vi "SDCCB Device Engine.vi"(0 "SDCCB Notifier Name":string="Box01", 11 "COM Port":string[](array[string])) -> ()   [LabVIEW 2020]
uses:
  Spinning Disk Type Defs/SD Notifer Data.ctl
  Spinning Disk Type Defs/SD Actions.ctl
  <vilib>/Instr/_visa.llb/VISA Configure Serial Port (Instr).vi
panel:
  in  "Get All Positions":bool
  in  "Disk On":bool
  in  "Disk Position":i32=1 min=1 max=3
  out "Latest Error":errorcluster
  in  "Quit":bool
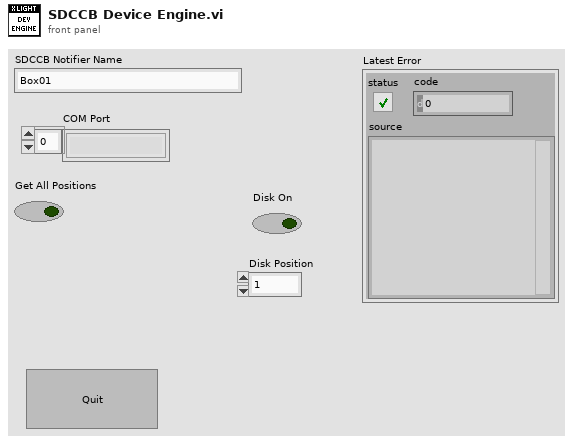
[diagram p1: front panel]
types:
  T1 = typedef "SD Notifer Data.ctl" = cluster{"Actions":T2, "Disk On?":bool, "Dichroic Pos.":i32, "Filter Wheel Pos.":i32, "Disk Pos.":i32, "Recived":bool, "Num Pos":i32[]}
  T2 = typedef "SD Actions.ctl" = enum16{"Status", "Get All Pos.", "Get Num. Pos.", "Home All", "Set Filter Wheel Pos.", "Set Disk Pos.", "Set Dichroic Pos.", "Disk On", "Disk Off", "Quit"}
  T3 = enum32{"Invalid", "Standard", "Closed", "Hidden", "Minimized", "Maximized"}
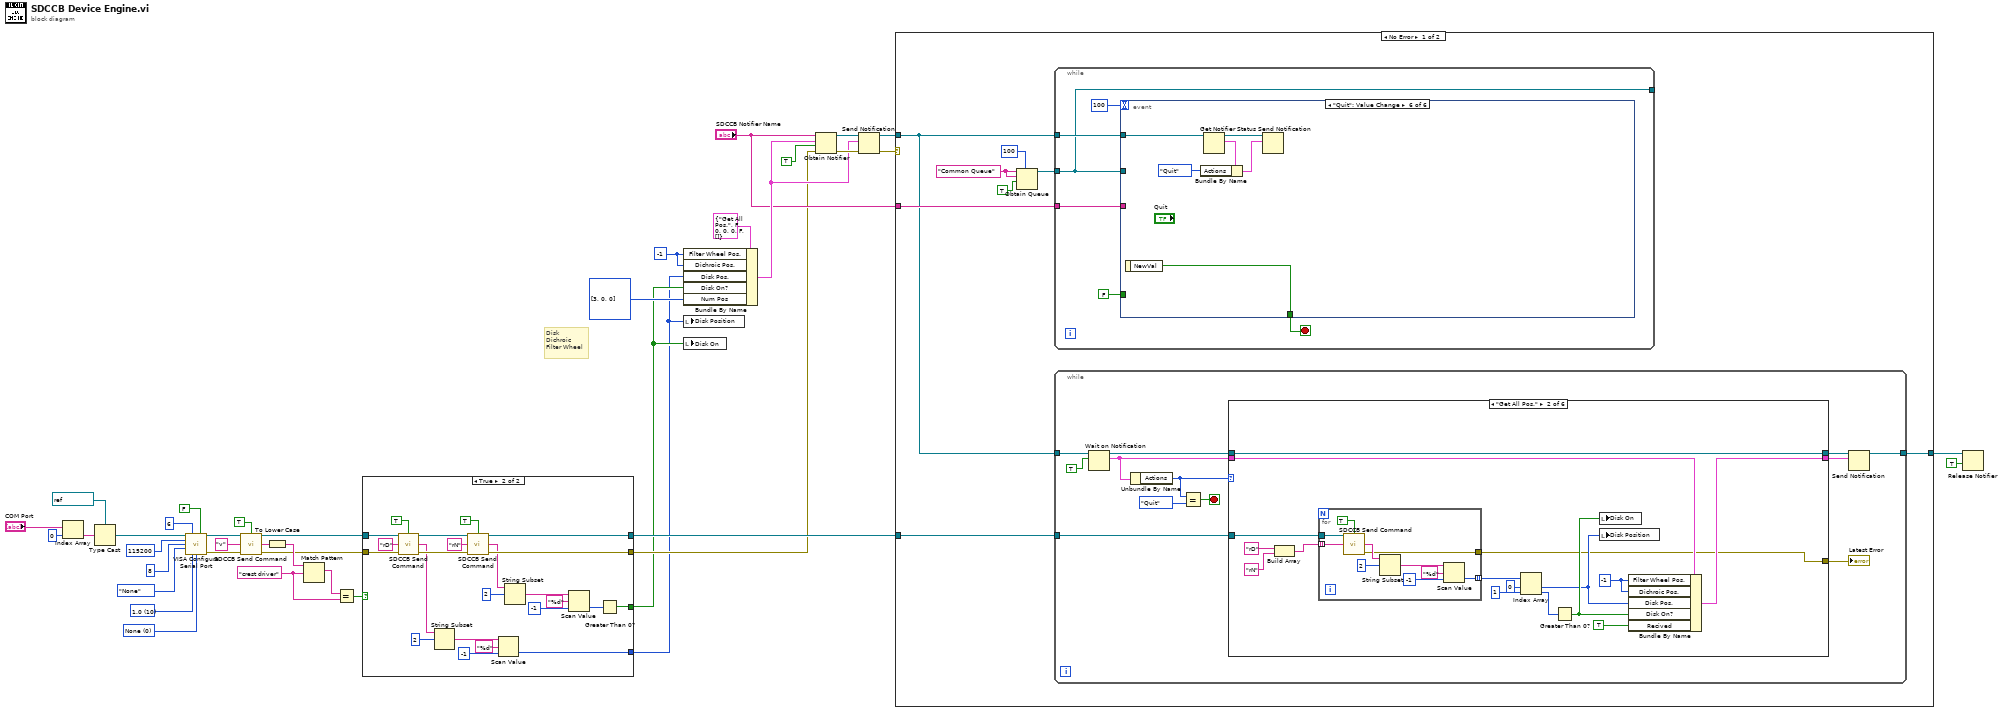
[diagram p0: block diagram]
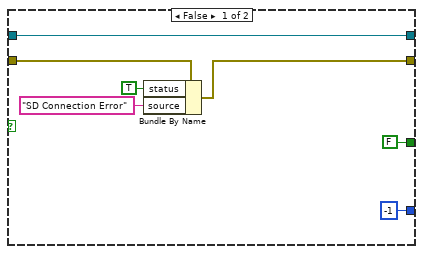
[diagram p2: hidden frame]
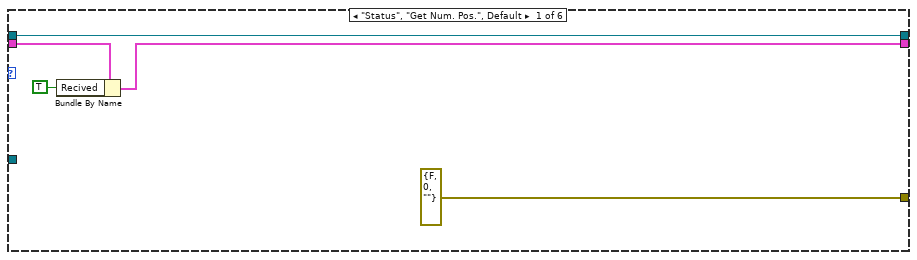
[diagram p3: hidden frame]
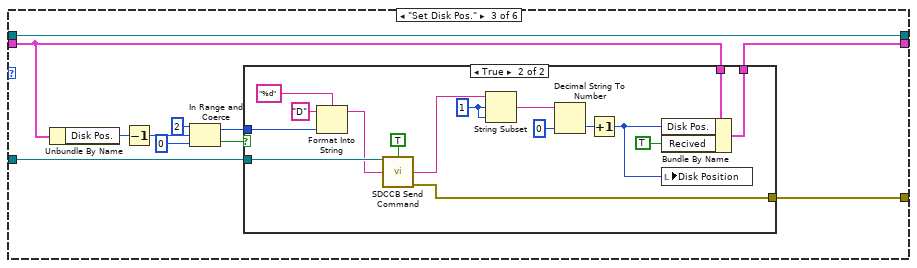
[diagram p4: hidden frame]
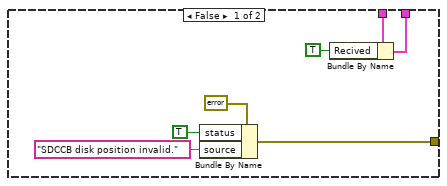
[diagram p5: hidden frame]
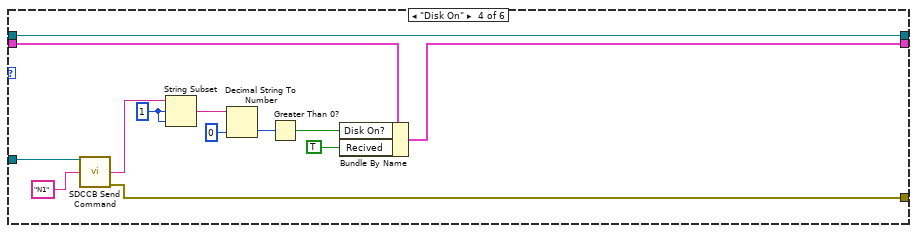
[diagram p6: hidden frame]
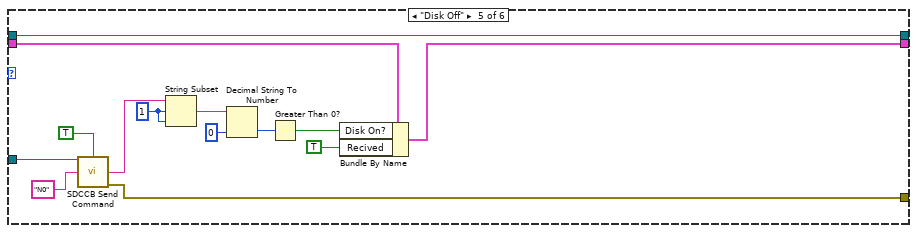
[diagram p7: hidden frame]
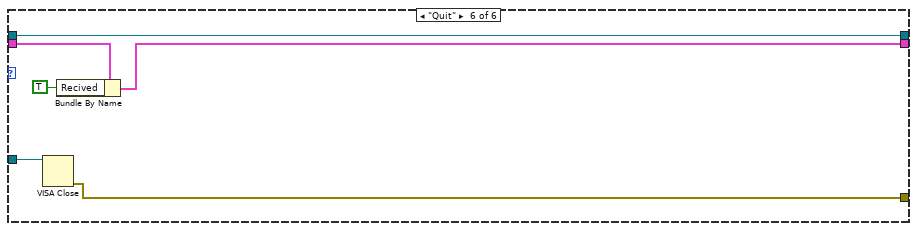
[diagram p8: hidden frame]
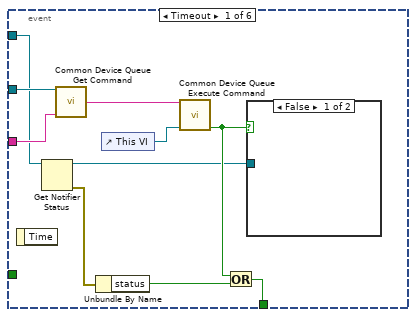
[diagram p9: hidden frame]
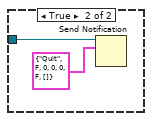
[diagram p10: hidden frame]
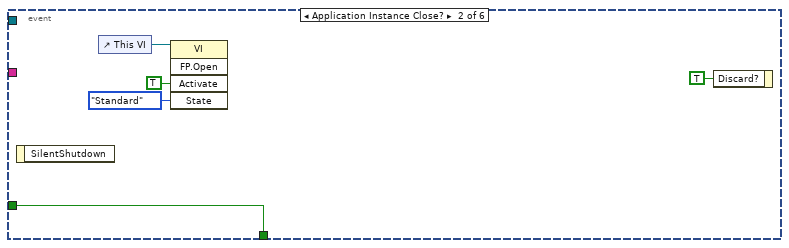
[diagram p11: hidden frame]
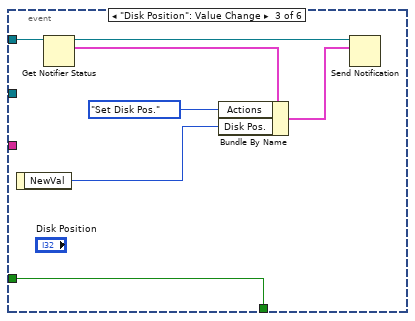
[diagram p12: hidden frame]
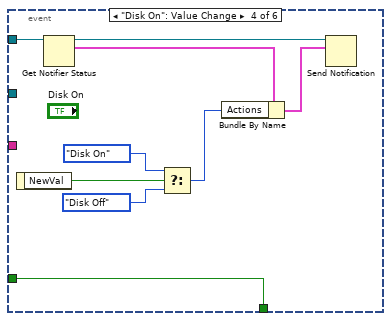
[diagram p13: hidden frame]
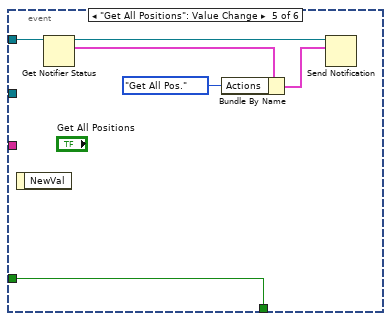
[diagram p14: hidden frame]
diagram:
  w10 = "crest driver"
  w13 = -1 ("Filter Wheel Pos.")
  w18 = u16 0 items=["None", "XON/XOFF", "RTS/CTS", "XON/XOFF & RTS/CTS", "DTR/DSR", "XON/XOFF & DTR/DSR"] ("flow control (0:none)")
  w19 = u16 10 items=["1.0"=10, "1.5"=15, "2.0"=20] ("stop bits (10: 1 bit)")
  # "Disk\nDichroic\nFilter Wheel"
  n1 = Index Array(array="COM Port", index=0) -> (element=w36:string)
  n2 = Type Cast(type=refnum<visa-resource-name> "COM5" ("VISA resource name"), x=w36) -> (*(type *) &x=w16:refnum<visa-resource-name>)
  n3 = call-poly "VISA Configure Serial Port"("VISA resource name"=w16, "timeout (10sec)"=u32 6, "Enable Termination\nChar (T)"=FALSE ("Enable Termination\nChar (T)"), "baud rate (9600)"=u32 115200, "data bits (8)"=u16 8, "parity (0:none)"=enum16{"None", "Odd", "Even", "Mark", "Space"}."None", "stop bits (10: 1 bit)"=w19, "flow control (0:none)"=w18) -> ("VISA resource name out"=w15:refnum<visa-resource-name>, "error out"=w14:errorcluster)  [unwired: 6 in]
  n4 = call "SDCCB Send Command.vi"("VISA Ref"=w15, "Wait for Reply (T)"=TRUE, "Command"="v", "Error In"=w14) -> ("VISA Ref Dup"=w6:refnum<visa-resource-name>, "Reply"=w9:string, "Error Out"=w7:errorcluster)  [unwired: 9 in]
  n5 = To Lower Case(string=w9) -> (all lower case string=w12:string)
  n6 = Match Pattern(string=w12, regular expression=w10) -> (match substring=w11:string)  [unwired: 1 in, 3 out]
  n7 = Equal?(x=w11, y=w10) -> (x = y?=w8:bool)
  n8 = case shown="True" w8 {
    tunnel: w7 -> [w46 w67]
    tunnel: [w43 w61] -> w3
    tunnel: w6 -> [w42 w69]
    tunnel: [w42 w49] -> w4
    tunnel: [FALSE w48] -> w2
    tunnel: [-1 ("default (0 dbl)") w47] -> w1
    frame False {
      n9 = Bundle By Name(cluster=w46, "status"=TRUE, "source"="SD Connection Error") -> (w43:errorcluster)
    }
    frame True {
      n10 = call "SDCCB Send Command.vi"("VISA Ref"=w69, "Wait for Reply (T)"=TRUE, "Command"="rD", "Error In"=w67) -> ("VISA Ref Dup"=w62:refnum<visa-resource-name>, "Reply"=w60:string, "Error Out"=w63:errorcluster)  [unwired: 9 in]
      n11 = String Subset(string=w60, offset (0)=2) -> (substring=w58:string)  [unwired: 1 in]
      n12 = call "SDCCB Send Command.vi"("VISA Ref"=w62, "Wait for Reply (T)"=TRUE, "Command"="rN", "Error In"=w63) -> ("VISA Ref Dup"=w49:refnum<visa-resource-name>, "Reply"=w51:string, "Error Out"=w61:errorcluster)  [unwired: 9 in]
      n13 = Scan Value(string=w58, format string="%d", default (0 dbl)=-1) -> (value=w47:i32)  [unwired: 1 out]
      n14 = String Subset(string=w51, offset (0)=2) -> (substring=w53:string)  [unwired: 1 in]
      n15 = Scan Value(string=w53, format string="%d", default (0 dbl)=-1) -> (value=w50:i32)  [unwired: 1 out]
      n16 = Greater Than 0?(x=w50) -> (x > 0?=w48:bool)
    }
  }
  n17 = Bundle By Name(cluster=T1 {"Actions"=enum."Get All Pos.", "Disk On?"=FALSE, "Dichroic Pos."=0, "Filter Wheel Pos."=0, "Disk Pos."=0, "Recived"=FALSE, "Num Pos"=[]} ("XLight Notifier Data"), "Filter Wheel Pos."=w13, "Dichroic Pos."=w13, "Disk Pos."=w1, "Disk On?"=w2, "Num Pos"=i32[] [3, 0, 0]) -> (w30:T1)
  n18 = local write "Disk Position"(w1) -> ()
  n19 = local write "Disk On"(w2) -> ()
  n20 = Obtain Notifier(name (unnamed)="SDCCB Notifier Name", notification data type=w30, create if not found? (T)=TRUE, error in (no error)=w3) -> (notifier out=w34:refnum<notifier>, error out=w33:errorcluster)  [unwired: 1 out]
  n21 = Send Notification(notification=w30, notifier=w34, error in (no error)=w33) -> (notifier out=w28:refnum<notifier>, error out=w29:errorcluster)
  n22 = case shown="No Error" w29 {
    tunnel: w28 -> [w71 w239]
    tunnel: w4 -> [w72 _]
    tunnel: "SDCCB Notifier Name" -> [w77 _]
    tunnel: [w70 w239] -> w26
    frame No Error {
      w76 = "Common Queue" ("Unique Notifier Name")
      n23 = Obtain Queue(max queue size (-1, unlimited)=100, name (unnamed)=w76, element data type=w76, create if not found? (T)=TRUE) -> (queue out=w73:refnum<queue>)  [unwired: 1 in, 2 out]
      n24 = while {
        tunnel: w73 -> [w188]
        tunnel: w77 -> [w191]
        tunnel: w71 -> [w192]
        tunnel: [w188] -> _
        stop <- w190 stop-if-true
        # "ProScan 3 GUI and Common Queue Loop"
        n25 = event shown="[5] \"Quit\": Value Change" {
          selector: _ -> [_ _ _ _ _ _]
          dyn-events: _ -> [_ _ _ _ _ _]
          timeout: 100 -> [_ _ _ _ _ _]
          tunnel: w188 -> [w197 _ _ _ _ _]
          tunnel: w192 -> [w194 _ w216 w225 w231 w237]
          tunnel: w191 -> [w196 _ _ _ _ _]
          tunnel: [w195 w210 w217 w226 w232 w238] -> w190
          tunnel: FALSE -> [_ w210 w217 w226 w232 _]
          event Timeout {
            n26 = event-data() -> ()  [unwired: 1 in, 1 out]
            n27 = Get Notifier Status(notifier=w194) -> (notifier out=w198:refnum<notifier>, error out=w203:errorcluster)  [unwired: 1 in, 3 out]
            n28 = call "Common Device Queue Get Command.vi"("Common Queue"=w197, "Notifier Name"=w196) -> ("Command"=w202:string)  [unwired: 12 in, 1 out]
            n29 = Unbundle By Name(w203) -> ("status"=w200:bool)
            n30 = control-ref of="This VI"() -> (w201:refnum<vi>)
            n31 = call "Common Device Queue Execute Command.vi"("Common Command"=w202, "VI Refnum"=w201) -> ("Quit?"=w199:bool)  [unwired: 12 in, 1 out]
            n32 = Or(x=w199, y=w200) -> (x .or. y?=w195:bool)
            n33 = case shown="False" w199 {
              tunnel: w198 -> [_ w205]
              frame False {
              }
              frame True {
                n34 = Send Notification(notification=T1 {"Actions"=enum."Quit", "Disk On?"=FALSE, "Dichroic Pos."=0, "Filter Wheel Pos."=0, "Disk Pos."=0, "Recived"=FALSE, "Num Pos"=[]} ("XLight Notifier Data"), notifier=w205) -> ()  [unwired: 1 in, 2 out]
              }
            }
          }
          event Application Instance Close? {
            n35 = event-data() -> ()  [unwired: 1 in, 1 out]
            n36 = control-ref of="This VI"() -> (w207:refnum<vi>)
            n37 = invoke class="VI" method="FP.Open"(reference=w207, "Activate"=TRUE ("Activate?"), "State"=T3."Standard") -> ()  [unwired: 2 in, 5 out]
            n38 = event-data("Discard?"=TRUE) -> ()  [unwired: 1 in, 1 out]
          }
          event "Disk Position": Value Change {
            n39 = event-data() -> ("NewVal"=w212:i32)  [unwired: 1 in]
            n40 = Get Notifier Status(notifier=w216) -> (notifier out=w215:refnum<notifier>, current notification=w214:T1)  [unwired: 1 in, 3 out]
            n41 = Bundle By Name(cluster=w214, "Actions"=SD_Actions."Set Disk Pos.", "Disk Pos."=w212) -> (w211:T1)
            n42 = Send Notification(notification=w211, notifier=w215) -> ()  [unwired: 1 in, 2 out]
          }
          event "Disk On": Value Change {
            n43 = event-data() -> ("NewVal"=w221:bool)  [unwired: 1 in]
            n44 = Get Notifier Status(notifier=w225) -> (notifier out=w224:refnum<notifier>, current notification=w223:T1)  [unwired: 1 in, 3 out]
            n45 = Select(t=SD_Actions."Disk On" ("Actions"), s=w221, f=SD_Actions."Disk Off" ("Actions")) -> (s? t:f=w218:T2)
            n46 = Bundle By Name(cluster=w223, "Actions"=w218) -> (w222:T1)
            n47 = Send Notification(notification=w222, notifier=w224) -> ()  [unwired: 1 in, 2 out]
          }
          event "Get All Positions": Value Change {
            n48 = event-data() -> ()  [unwired: 1 in, 1 out]
            n49 = Get Notifier Status(notifier=w231) -> (notifier out=w230:refnum<notifier>, current notification=w229:T1)  [unwired: 1 in, 3 out]
            n50 = Bundle By Name(cluster=w229, "Actions"=SD_Actions."Get All Pos.") -> (w228:T1)
            n51 = Send Notification(notification=w228, notifier=w230) -> ()  [unwired: 1 in, 2 out]
          }
          event "Quit": Value Change {
            n52 = event-data() -> ("NewVal"=w238:bool)  [unwired: 1 in]
            n53 = Get Notifier Status(notifier=w237) -> (notifier out=w234:refnum<notifier>, current notification=w236:T1)  [unwired: 1 in, 3 out]
            n54 = Bundle By Name(cluster=w236, "Actions"=SD_Actions."Quit") -> (w233:T1)
            n55 = Send Notification(notification=w233, notifier=w234) -> ()  [unwired: 1 in, 2 out]
          }
        }
      }
      n56 = while {
        tunnel: w72 -> [w80]
        tunnel: w71 -> [w89]
        tunnel: [w78] -> w70
        stop <- w86 stop-if-true
        n57 = Wait on Notification(notifier=w89, ignore previous (F)=TRUE) -> (notifier out=w84:refnum<notifier>, notification=w83:T1)  [unwired: 2 in, 2 out]
        n58 = Unbundle By Name(w83) -> ("Actions"=w85:T2)
        n59 = Equal?(x=w85, y=SD_Actions."Quit") -> (x = y?=w86:bool)
        n60 = case shown="\"Get All Pos.\"" w85 {
          tunnel: w84 -> [w94 w110 w131 w167 w181 w187]
          tunnel: w83 -> [w93 w109 w128 w164 w178 w186]
          tunnel: [w94 w110 w131 w167 w181 w187] -> w82
          tunnel: [w91 w107 w127 w158 w172 w184] -> w81
          tunnel: w80 -> [_ w102 w130 w166 w180 w183]
          tunnel: [errorcluster {"status"=FALSE, "code"=0, "source"=""} ("Error Out") w95 w129 w165 w179 w182] -> w79
          frame "Status", "Get Num. Pos.", Default {
            n61 = Bundle By Name(cluster=w93, "Recived"=TRUE) -> (w91:T1)
          }
          frame "Get All Pos." {
            w106 = -1 ("Filter Wheel Pos.")
            n62 = Build Array("rD" ("Command"), "rN" ("Command")) -> (w105:string[])
            n63 = for {
              tunnel: [w114] -> w101 mode=indexing
              tunnel: w105 -> [w113] mode=indexing
              tunnel: w102 -> [w112]
              tunnel: [w111] -> w95
              n64 = call "SDCCB Send Command.vi"("VISA Ref"=w112, "Wait for Reply (T)"=TRUE, "Command"=w113) -> ("Reply"=w119:string, "Error Out"=w111:errorcluster)  [unwired: 10 in, 1 out]
              n65 = String Subset(string=w119, offset (0)=2) -> (substring=w117:string)  [unwired: 1 in]
              n66 = Scan Value(string=w117, format string="%d", default (0 dbl)=-1) -> (value=w114:i32)  [unwired: 1 out]
            }
            n67 = Index Array(array=w101, index #1=0 ("index"), index #2=1 ("index")) -> (element #1=w96:i32, element #2=w98:i32)
            n68 = Greater Than 0?(x=w98) -> (x > 0?=w97:bool)
            n69 = local write "Disk On"(w97) -> ()
            n70 = local write "Disk Position"(w96) -> ()
            n71 = Bundle By Name(cluster=w109, "Filter Wheel Pos."=w106, "Dichroic Pos."=w106, "Disk Pos."=w96, "Disk On?"=w97, "Recived"=TRUE) -> (w107:T1)
          }
          frame "Set Disk Pos." {
            n72 = Unbundle By Name(w128) -> ("Disk Pos."=w126:i32)
            n73 = Decrement(x=w126) -> (x-1=w121:i32)
            n74 = In Range and Coerce(upper limit=2, x=w121, lower limit=0) -> (coerced(x)=w122:i32, In Range?=w123:bool)
            n75 = case shown="True" w123 {
              tunnel: w130 -> [_ w154]
              tunnel: [w132 w153] -> w129
              tunnel: w128 -> [w137 w149]
              tunnel: [w136 w143] -> w127
              tunnel: w122 -> [_ w142]
              frame False {
                n76 = Bundle By Name(cluster=errorcluster {"status"=FALSE, "code"=0, "source"=""} ("Error Out"), "status"=TRUE, "source"="SDCCB disk position invalid.") -> (w132:errorcluster)
                n77 = Bundle By Name(cluster=w137, "Recived"=TRUE) -> (w136:T1)
              }
              frame True {
                w146 = 1 ("offset (0)")
                n78 = Format Into String(format string="%d", initial string="D", w142) -> (resulting string=w150:string)  [unwired: 1 in, 1 out]
                n79 = call "SDCCB Send Command.vi"("VISA Ref"=w154, "Wait for Reply (T)"=TRUE, "Command"=w150) -> ("Reply"=w147:string, "Error Out"=w153:errorcluster)  [unwired: 10 in, 1 out]
                n80 = String Subset(string=w147, offset (0)=w146, length (rest)=w146) -> (substring=w145:string)
                n81 = Decimal String To Number(string=w145, default (0L)=0 ("default (0 I32)")) -> (number=w141:i32)  [unwired: 1 in, 1 out]
                n82 = Increment(x=w141) -> (x+1=w140:i32)
                n83 = Bundle By Name(cluster=w149, "Disk Pos."=w140, "Recived"=TRUE) -> (w143:T1)
                n84 = local write "Disk Position"(w140) -> ()
              }
            }
          }
          frame "Disk On" {
            w161 = 1 ("offset (0)")
            n85 = call "SDCCB Send Command.vi"("VISA Ref"=w166, "Command"="N1" ("initial string")) -> ("Reply"=w162:string, "Error Out"=w165:errorcluster)  [unwired: 11 in, 1 out]
            n86 = String Subset(string=w162, offset (0)=w161, length (rest)=w161) -> (substring=w160:string)
            n87 = Decimal String To Number(string=w160, default (0L)=0 ("default (0 I32)")) -> (number=w157:i32)  [unwired: 1 in, 1 out]
            n88 = Greater Than 0?(x=w157) -> (x > 0?=w156:bool)
            n89 = Bundle By Name(cluster=w164, "Disk On?"=w156, "Recived"=TRUE) -> (w158:T1)
          }
          frame "Disk Off" {
            w175 = 1 ("offset (0)")
            n90 = call "SDCCB Send Command.vi"("VISA Ref"=w180, "Wait for Reply (T)"=TRUE, "Command"="N0" ("initial string")) -> ("Reply"=w176:string, "Error Out"=w179:errorcluster)  [unwired: 10 in, 1 out]
            n91 = String Subset(string=w176, offset (0)=w175, length (rest)=w175) -> (substring=w174:string)
            n92 = Decimal String To Number(string=w174, default (0L)=0 ("default (0 I32)")) -> (number=w171:i32)  [unwired: 1 in, 1 out]
            n93 = Greater Than 0?(x=w171) -> (x > 0?=w170:bool)
            n94 = Bundle By Name(cluster=w178, "Disk On?"=w170, "Recived"=TRUE) -> (w172:T1)
          }
          frame "Quit" {
            n95 = VISA Close(VISA resource name=w183) -> (error out=w182:errorcluster)  [unwired: 1 in]
            n96 = Bundle By Name(cluster=w186, "Recived"=TRUE) -> (w184:T1)
          }
        }
        "Latest Error" <- w79
        n97 = Send Notification(notification=w81, notifier=w82) -> (notifier out=w78:refnum<notifier>)  [unwired: 1 in, 1 out]
      }
    }
    frame Error {
    }
  }
  n98 = Release Notifier(notifier=w26, force destroy? (F)=TRUE) -> ()  [unwired: 1 in, 3 out]
